vi "Send DisplayPopup_UI.vi"(7 "Message Priority (Normal)":T2=enum."Normal", 8 "error in (no error)":errorcluster, 10 "PopupDetails":T1, 11 "Message Enqueuer":refnum<class "Message Enqueuer.lvclass">) -> (0 "error out":errorcluster, 3 "Message Enqueuer out":refnum<class "Message Enqueuer.lvclass">)   [LabVIEW 2019, in "ZenGage v3.0 UI.lvlib" / "DisplayPopup_UI.lvclass"]
doc: "This VI sends the message to an actor."
uses:
  DisplayPopup_UI.lvclass
  <vilib>/ActorFramework/Message Enqueuer/Message Enqueuer.lvclass
  C:/Program Files/National Instruments/LabVIEW 2019/vi.lib/ActorFramework/Message/Message.lvclass
  <vilib>/ActorFramework/Message Enqueuer/Message Priority.ctl
  Common/Controls/Pop-up Input.ctl
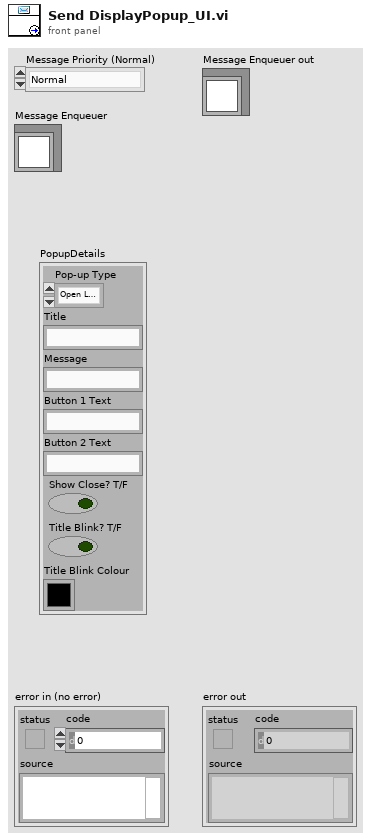
[diagram p1: front panel]
types:
  T1 = typedef "Pop-up Input.ctl" = cluster{"Pop-up Type":enum16{"Open Logo Display", "Close Logo Display", "Open Loading Bar", "Close Loading Bar", "Open Alert Display", "Close Alert Display", "One button dialog box", "Two button dialog box", "User Authentication"}, "Title":string, "Message":string, "Button 1 Text":string, "Button 2 Text":string, "Show Close? T/F":bool, "Title Blink? T/F":bool, "Title Blink Colour":u32}
  T2 = typedef "Actor Framework.lvlib/Message Enqueuer.lvclass/Message Priority.ctl" = enum16{"Low", "Normal", "High"}
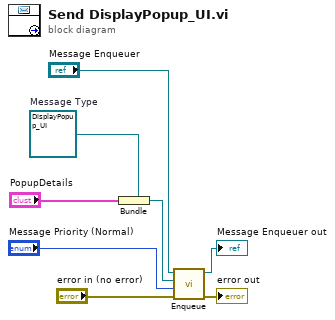
[diagram p0: block diagram]
diagram:
  w5 = refnum<class "DisplayPopup_UI.lvclass"> refnum  # Message Type
  n1 = Bundle(cluster=w5, "PopupDetails") -> (w4:refnum<class "DisplayPopup_UI.lvclass">)
  n2 = call <vilib>:"Enqueue.vi"("error in (no error)"="error in (no error)", "Message Priority (Normal)"="Message Priority (Normal)", "Message"=w4, "Message Enqueuer in"="Message Enqueuer") -> ("error out"=→"error out":errorcluster, "Message Enqueuer out"=→"Message Enqueuer out":refnum<class "Message Enqueuer.lvclass">)  [unwired: 6 in]
